vi "_DServerDisableStateMachine.vi"(2 "error in":errorcluster, 3 "device name":string="unspecified_device_name") -> (0 "error out":errorcluster)   [LabVIEW 2014, in "tango.lvlib"]
uses:
  tango.lvlib
  tango_binding.so
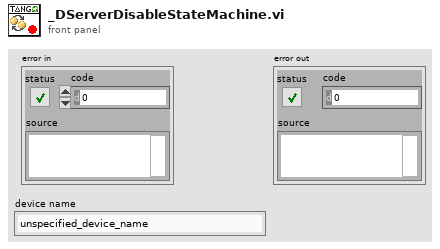
[diagram p1: front panel]
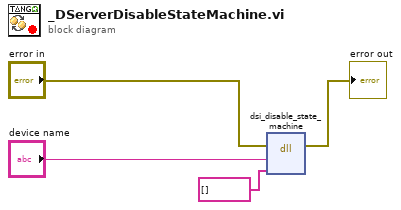
[diagram p0: block diagram]
diagram:
  n1 = dll-call lib="tango_binding.*" fn="dsi_disable_state_machine"(error in="error in", "device_name"="device name", "error_stack"=string[] [] ("error stack")) -> (error out=→"error out":errorcluster)  [unwired: 5 in, 1 out]
